vi "Get 2-Rayleigh Parameters (SubVI).vi"(6 "Flow Peak Amp.":dbl, 8 "T_Flow Start (s)":dbl, 9 "T_Flow Peak (s)":dbl, 10 "T_Ejection period (s)":dbl, 11 "Pressure (mmHg)":waveform(dbl)) -> (3 "Optimised Parameter":dbl[](array[numeric]))   [LabVIEW 2017]
uses:
  72fe1329-4430-4fd7-86c8-dfab2f7b2d2e.vi
  5c84d562-1cd3-438d-9587-7d7d9e0fcbf7.vi
panel:
  out "Waveform Graph":waveform(dbl)(graph)
  out "appended array":dbl[](array[numeric])
  out "Logic":bool
  out "Numeric 2":i32
  out "Numeric":i32
  out "sorted 2D array":dbl[][](array[numeric])
  out "x-1":i32
  out "sorted array of params":dbl[][](array[numeric])
  out "Error Checks":dbl[][](array[numeric])
  out "Parameters":dbl[][](array[numeric])
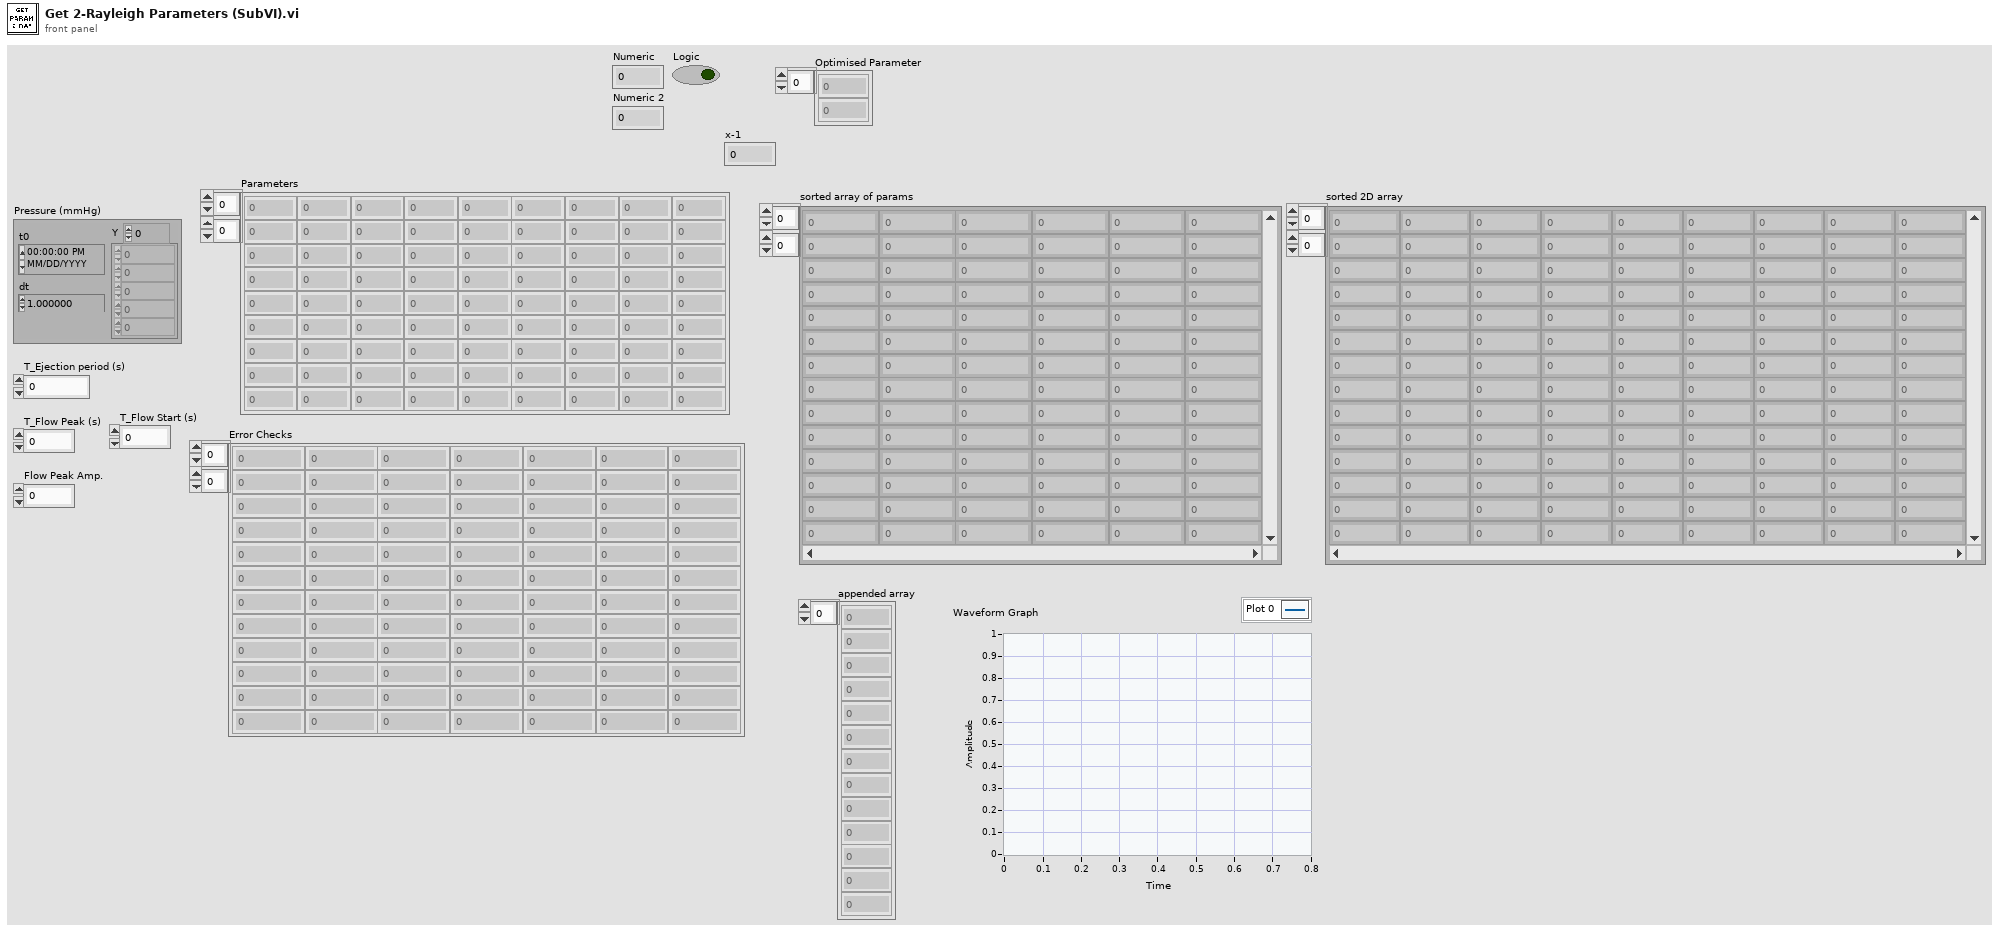
[diagram p1: front panel]
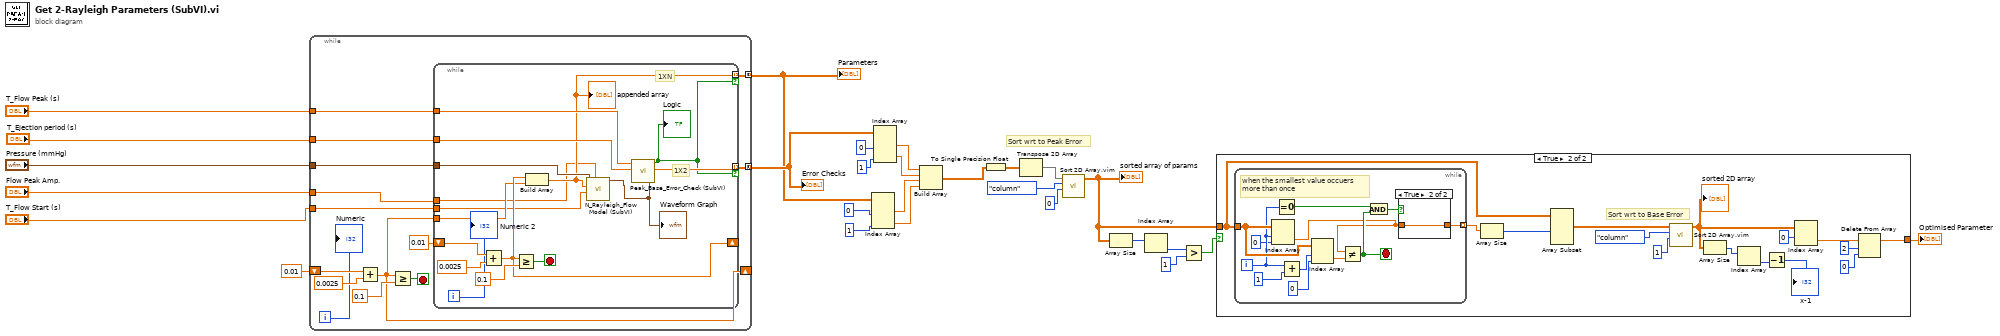
[diagram p0: block diagram]
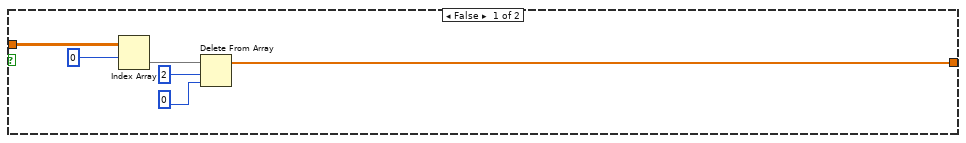
[diagram p2: hidden frame]
diagram:
  # "Sort wrt to Peak Error"
  n1 = while {
    tunnel: "Pressure (mmHg)" -> [w41]
    tunnel: "Flow Peak Amp." -> [w40]
    shift-right: [w35] -> _
    shift-left: 0.01 ("start") -> [w38]
    tunnel: "T_Ejection period (s)" -> [w33]
    tunnel: "T_Flow Peak (s)" -> [w32]
    tunnel: [w31] -> w12 mode=concatenating
    tunnel: [w30] -> w17 mode=concatenating
    tunnel: "T_Flow Start (s)" -> [w29]
    i -> [w28]
    stop <- w36 stop-if-true
    n2 = Add(x=w38, y=0.0025 ("start")) -> (x+y=w35:dbl)
    n3 = Greater Or Equal?(x=w35, y=0.1 ("start")) -> (x >= y?=w36:bool)
    n4 = while {
      tunnel: w41 -> [w46]
      tunnel: w40 -> [w43]
      tunnel: w35 -> [w48]
      shift-right: [w49] -> _
      shift-left: 0.01 ("start") -> [w55]
      tunnel: w33 -> [w53]
      tunnel: w32 -> [w52]
      tunnel: [w44] -> w31 mode=indexing if=w50
      tunnel: [w51] -> w30 mode=indexing if=w50
      tunnel: w29 -> [w45]
      i -> [w47]
      stop <- w54 stop-if-true
      # "1X2"
      # "1XN"
      n5 = Add(x=w55, y=0.0025 ("start")) -> (x+y=w49:dbl)
      n6 = Greater Or Equal?(x=w49, y=0.1 ("start")) -> (x >= y?=w54:bool)
      n7 = Build Array(w49, w48) -> (w44:dbl[])
      "appended array" <- w44
      n8 = call "N_Rayleigh_Flow Model (SubVI).vi"("PSQ (ml/s)"=w43, "T_Flow Start"=w45, "Parameters (1XN)"=w44, "Pressure (mmHg)"=w46) -> ("n-Rayleigh Model Flow"=w42:waveform(dbl))  [unwired: 4 in, 1 out]
      "Waveform Graph" <- w42
      n9 = call "Peak_Base_Error_Check (SubVI).vi"("Model Flow"=w42, "T_Ejection Period (s)"=w53, "T_Flow Peak (s)"=w52) -> ("Error"=w51:dbl[], "Logic"=w50:bool)  [unwired: 5 in, 2 out]
      "Logic" <- w50
      "Numeric 2" <- w47
    }
    "Numeric" <- w28
  }
  "Parameters" <- w12
  "Error Checks" <- w17
  n10 = Index Array(array=w12, index (col) #1=0 ("disabled index (col)"), index (col) #2=1 ("index (col)")) -> (element #1=w14:dbl[], element #2=w13:dbl[])  [unwired: 2 in]
  n11 = Index Array(array=w17, index (col) #1=0 ("disabled index (col)"), index (col) #2=1 ("index (col)")) -> (element #1=w16:dbl[], element #2=w15:dbl[])  [unwired: 2 in]
  n12 = Build Array(w16, w15, w14, w13) -> (w3:dbl[][])
  n13 = To Single Precision Float(number=w3) -> (single precision float=w4:sgl[][])
  n14 = Transpose 2D Array(2D array=w4) -> (transposed array=w11:sgl[][])
  n15 = call "Sort 2D Array.vim"("index"=0, "dimension to index (column)"=enum16{"column", "row"}."column", "2D array"=w11) -> ("sorted 2D array"=w5:sgl[][])  [unwired: 7 in, 1 out]
  "sorted array of params" <- w5
  n16 = Array Size(array=w5) -> (size(s)=w9:i32[])
  n17 = Index Array(array=w9) -> (element=w8:i32)  [unwired: 1 in]
  n18 = Greater?(x=w8, y=1) -> (0:w7:bool)
  n19 = case shown="True" w7 {
    tunnel: w5 -> [w63 w67]
    tunnel: [w58 w66] -> w6
    frame False {
      n20 = Index Array(array=w63, index (row)=0) -> (element=w61:sgl[])  [unwired: 1 in]
      n21 = Delete From Array(array=w61, length=2, index=0) -> (array with subset deleted=w58:sgl[])  [unwired: 1 out]
    }
    frame True {
      # "Sort wrt to Base Error"
      n22 = while {
        tunnel: w67 -> [w88]
        tunnel: [w85] -> w68 mode=indexing
        i -> [w87]
        stop <- w81 stop-if-true
        # "when the smallest value occuers \nmore than once"
        n23 = Index Array(array=w88, index (row)=w87, index (col)=0 ("disabled index (col)")) -> (element=w80:sgl)
        n24 = Equal To 0?(x=w87) -> (x = 0?=w86:bool)
        n25 = Add(x=w87, y=1) -> (x+y=w89:i32)
        n26 = Index Array(array=w88, index (row)=w89, index (col)=0 ("disabled index (col)")) -> (element=w79:sgl)
        n27 = Not Equal?(x=w80, y=w79) -> (x != y?=w81:bool)
        n28 = And(x=w86, y=w81) -> (x .and. y?=w82:bool)
        n29 = case shown="True" w82 {
          tunnel: w80 -> [w91 w92]
          tunnel: [w91 w92] -> w85
          frame False {
          }
          frame True {
          }
        }
      }
      n30 = Array Size(array=w68) -> (size(s)=w65:i32)
      n31 = Array Subset(array=w67, length (row)=w65) -> (w73:sgl[][])  [unwired: 3 in]
      n32 = call "Sort 2D Array.vim"("index"=1, "dimension to index (column)"=enum16{"column", "row"}."column", "2D array"=w73) -> ("sorted 2D array"=w74:sgl[][])  [unwired: 7 in, 1 out]
      "sorted 2D array" <- w74
      n33 = Array Size(array=w74) -> (size(s)=w75:i32[])
      n34 = Index Array(array=w75) -> (element=w76:i32)  [unwired: 1 in]
      n35 = Decrement(x=w76) -> (x-1=→"x-1":i32)
      n36 = Index Array(array=w74, index (row)=0) -> (element=w78:sgl[])  [unwired: 1 in]
      n37 = Delete From Array(array=w78, length=2, index=0) -> (array with subset deleted=w66:sgl[])  [unwired: 1 out]
    }
  }
  "Optimised Parameter" <- w6
